vi "SampleDependentMethod.vi"(8 "error in (no error)":errorcluster, 11 "SampleDependentLib in":refnum<class "SampleDependentLib.lvclass">) -> (0 "error out":errorcluster, 3 "SampleDependentLib out":refnum<class "SampleDependentLib.lvclass">)   [LabVIEW 2019, in "SampleDependentLibPPL.lvlib" / "SampleDependentLib.lvclass"]
uses:
  SampleDependentLib.lvclass
  obj/SampleProjectTargets/My Computer/ExtDependency.lvlibp/ExternalDepClass/ExternalDepClass.lvclass
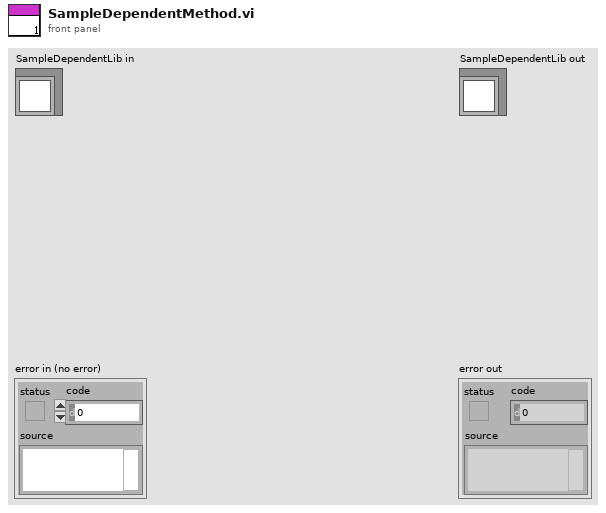
[diagram p1: front panel]
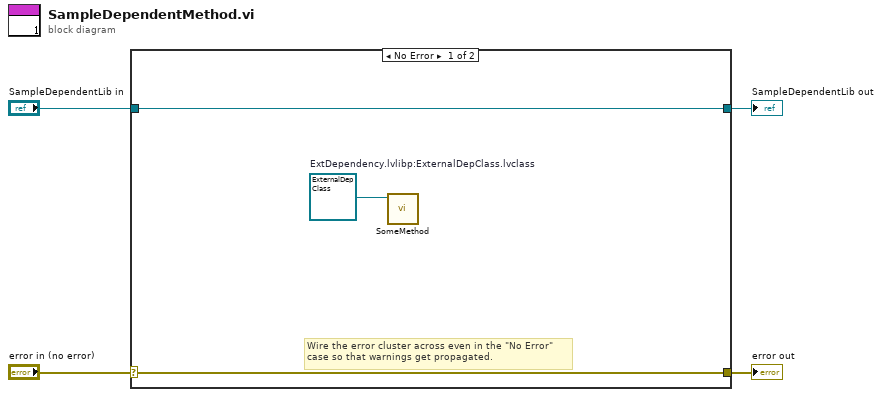
[diagram p0: block diagram]
diagram:
  n1 = case shown="No Error" "error in (no error)" {
    selector: "error in (no error)" -> [w6 w9]
    tunnel: [w6 w9] -> w3
    tunnel: [w7 w8] -> w1
    tunnel: "SampleDependentLib in" -> [w7 w8]
    frame No Error {
      w5 = refnum<class "ExternalDepClass.lvclass"> refnum  # ExtDependency.lvlibp:ExternalDepClass.lvclass
      # "Wire the error cluster across even in the \"No Error\"\ncase so that warnings get propagated."
      n2 = call-dynamic "SomeMethod.vi"("ExternalDepClass in"=w5) -> ()  [unwired: 9 in, 2 out]
    }
    frame Error {
    }
  }
  "error out" <- w3
  "SampleDependentLib out" <- w1
